vi "harp_connection_close.vi"(0 "port in":refnum<visa-resource-name>, 11 "error in":errorcluster) -> ()   [LabVIEW 2010]
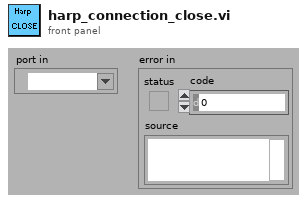
[diagram p1: front panel]
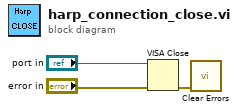
[diagram p0: block diagram]
diagram:
  n1 = VISA Close(VISA resource name="port in", error in (no error)="error in") -> (error out=w1:errorcluster)
  n2 = call <vilib>:"Clear Errors.vi"("error in (no error)"=w1) -> ()  [unwired: 6 in, 1 out]
